vi "Robot Global Data.vi"() -> ()   [LabVIEW 2020]
doc: "This global VI can contain as many global variables as you need. Place a control on the panel, give it a good name. To read or write to it from a VI, drag the icon to the diagram of that VI. You can also drag from the project. Click on the node to change which global you access. You shouldn't have multiple locations writing to a global or it will cause a race-condition."
uses:
  <vilib>/Rock Robotics/WPI/Camera/WPI_CameraImageSize.ctl
  <vilib>/Rock Robotics/WPI/DriverStation/WPI_DriverStationRobotMode2.ctl
panel:
  in  "Real Yaw":dbl
  out "Right Drive Encoder":dbl
  out "Left Drive Encoder":dbl
  in  "Target Blue":dbl
  in  "Target Red":dbl
  in  "Target Y":dbl
  in  "Target X":dbl
  in  "Red Arm Length":dbl=48.25
  out "Numeric 2":dbl
  in  "Blue Arm Length":dbl=38.125
  in  "Blue Lower limit":dbl
  in  "Red Lower limit":dbl
  in  "Blue higher limit":dbl=67.0
  in  "Red Higher limit":dbl=199.0
  in  "Small Farther Standerd X limit":dbl=30.5
  in  "Small Lower Standerd Y limit":dbl=-3.0
  in  "Closer Standerd X limit":dbl=19.0
  in  "Farther Standerd X limit":dbl=73.0
  in  "Lower Standerd Y limit":dbl=-8.0
  in  "Upper Standerd Y limit":dbl=66.0
  out "Blue Arm Limit Switch":bool
  out "zeroarmred":dbl
  out "zeroarmblue 2":dbl
  out "zeroarmblue":dbl
  out "Right High":dbl
  out "Right Low":dbl
  out "Left Low":dbl
  out "Left High":dbl
  out "Arm Red":dbl
  out "Arm Blue2":dbl
  out "Arm Blue":dbl
  in  "Game piece":dbl
  out "Arm Mode":bool
  in  "Pitch":dbl
  out "Last time":dbl
  out "Previose yaw":dbl
  out "Gyro Starting Value in our match":dbl
  out "yaw":dbl
  in  "Robot Mode":T1
  in  "image size":T2=enum."320x240"
  in  "Enable Vision":bool
  # "Encoder Values"
  # "Robot exclusion zone"
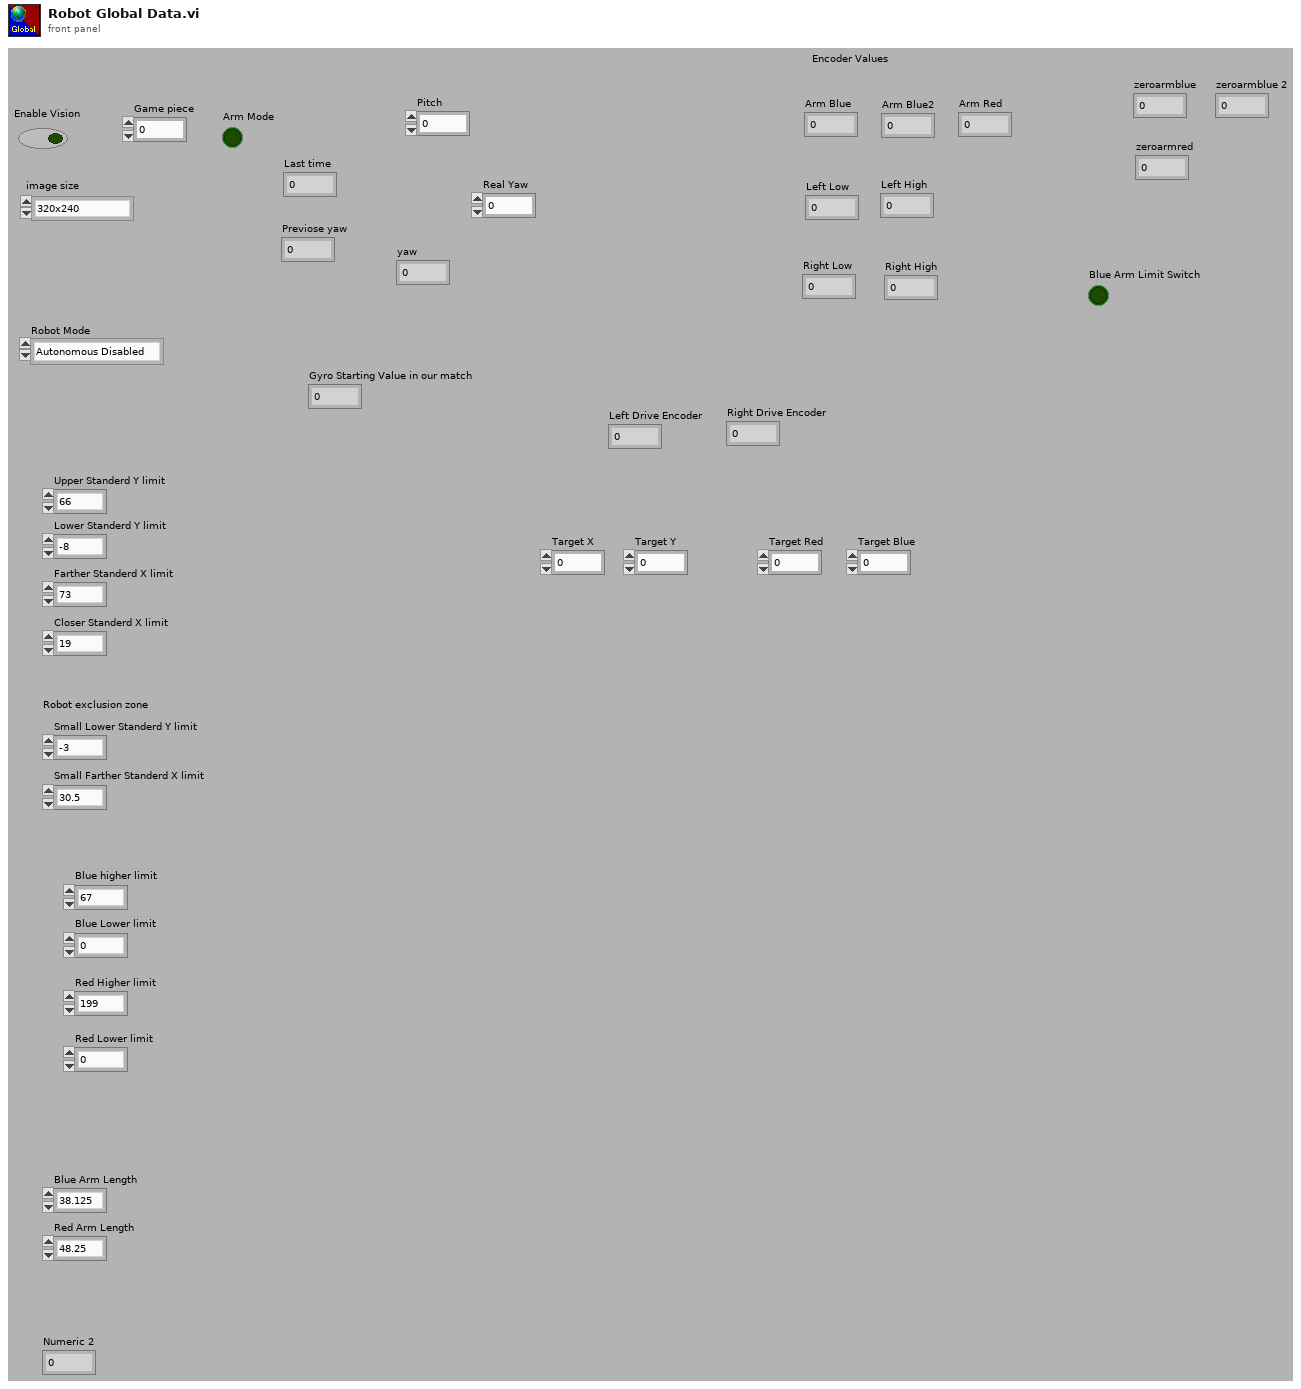
[diagram p1: front panel]
types:
  T1 = typedef "WPI_DriverStationRobotMode2.ctl" = enum16{"Autonomous Disabled", "Autonomous Enabled", "Teleop Disabled", "Teleop Enabled", "Disconnected", "Finish", "Test Disabled", "Test Enabled", "Emergency Stopped"}
  T2 = typedef "WPI_CameraImageSize.ctl" = enum16{"640x480", "320x240", "160x120", "Custom"}
diagram:
